vi "Find Visa Recorders.vi"(8 "Error In":errorcluster) -> (0 "Error Out":errorcluster, 2 "Names":string[](array[string]), 3 "Recorders List":refnum<class "Instrument Actor.lvclass">[](array[class]))   [LabVIEW 2019]
uses:
  Instrument Actor/Instrument Actor.lvclass
  <vilib>/Instr/_visa.llb/VISA Find Search Mode.ctl
panel:
  out "find list":refnum<visa-resource-name>[](array[refnum])
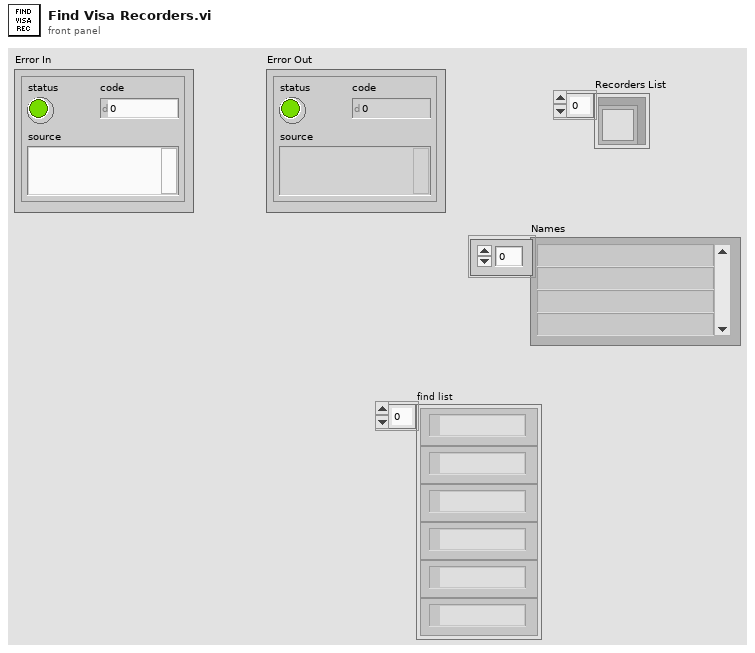
[diagram p1: front panel]
types:
  T1 = typedef "VISA Find Search Mode.ctl" = u32
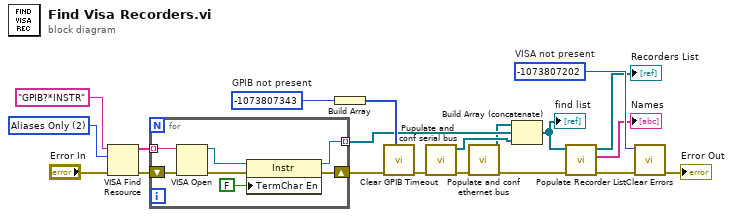
[diagram p0: block diagram]
diagram:
  w10 = -1073807202  # VISA not present
  w17 = -1073807343  # GPIB not present
  w19 = T1 2 items=["Canonical Names Only"=0, "Aliases Only"=2, "Include Matching Aliases"=3, "Include All Aliases"=4] ("Search Mode")
  n1 = VISA Find Resource(8:"Error In", 10:w19, 11:"GPIB?*INSTR" ("expression (\"?*\")")) -> (0:w14:errorcluster, 3:w12:string[])  [unwired: 1 out]
  n2 = for {
    shift-right: [w23] -> w13
    shift-left: w14 -> [w25]
    tunnel: w12 -> [w27] mode=indexing
    tunnel: [w22] -> w11 mode=indexing
    n3 = VISA Open(error in (no error)=w25, VISA resource name=w27) -> (VISA resource name=w26:refnum<visa-resource-name>, error out=w24:errorcluster)  [unwired: 3 in]
    n4 = property class="Instr"(reference=w26, error in=w24, "TermChar En"=FALSE ("Message Based Settings:Termination Character Enable")) -> (reference out=w22:refnum<visa-resource-name>, error out=w23:errorcluster)
  }
  n5 = Build Array(w17) -> (w16:i32[])
  n6 = call "Clear GPIB Timeout.vi"("Errors to skip"=w16, "error in (no error)"=w13) -> ("error out"=w15:errorcluster)  [unwired: 9 out]
  n7 = call "Pupulate and conf serial bus.vi"("Error In"=w15) -> ("Error Out"=w3:errorcluster, "Devices"=w18:refnum<visa-resource-name>[])  [unwired: 9 in]
  n8 = call "Populate and conf ethernet bus.vi"("Error In"=w3) -> ("Error Out"=w2:errorcluster, "Devices"=w1:refnum<visa-resource-name>[])  [unwired: 9 in]
  n9 = Build Array (concatenate)(w1, w11, w18) -> (w7:refnum<visa-resource-name>[])
  "find list" <- w7
  n10 = call "Populate Recorder List.vi"("error in (no error)"=w2, "VISA Resourse Names"=w7) -> ("error out"=w6:errorcluster, "Names"=→"Names":string[], "Instrument List"=→"Recorders List":refnum<class "Instrument Actor.lvclass">[])  [unwired: 7 in]
  n11 = call <vilib>:"Clear Errors.vi"("error in (no error)"=w6, "specific error code to clear (0: all)"=w10) -> ("error out"=→"Error Out":errorcluster)  [unwired: 4 in, 1 out]
